vi "Day 4 Puzzle 1.vi"(11 "Path":path) -> ()   [LabVIEW 2021]
uses:
  <vilib>/Utility/file.llb/Read Delimited Spreadsheet (string).vi
panel:
  out "Number of contained":i32
  out "Array 4":bool[](array[boolean])
  out "Elf 2":i32[][](array[numeric])
  out "Elf 1":i32[][](array[numeric])
  out "subarray":string[](array[string])
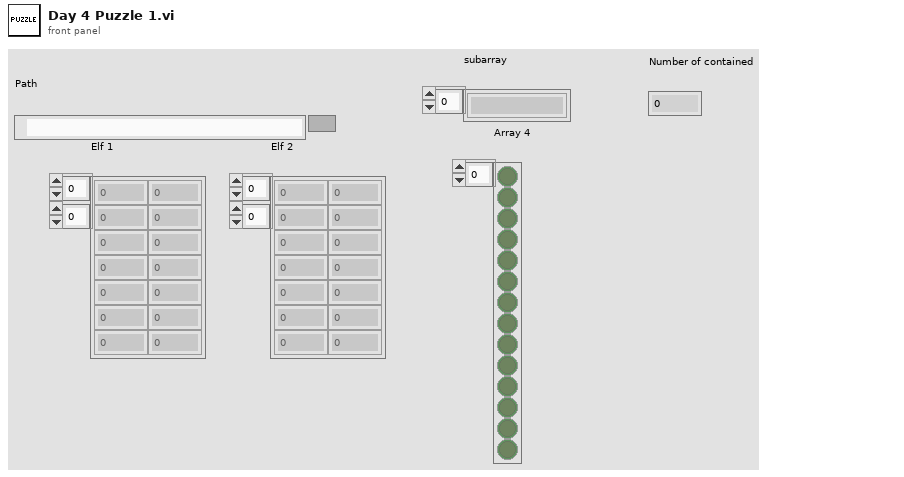
[diagram p1: front panel]
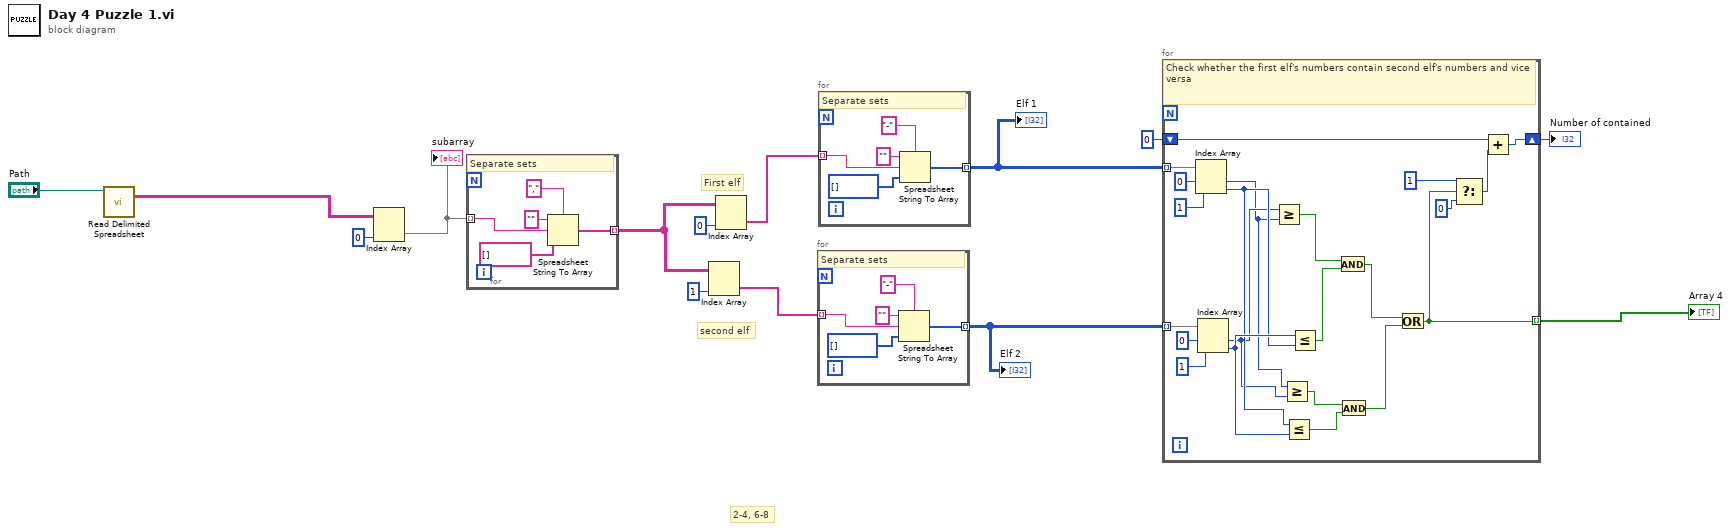
[diagram p0: block diagram]
diagram:
  # "2-4, 6-8"
  # "second elf"
  # "First elf"
  n1 = call-poly <vilib>:"Read Delimited Spreadsheet.vi"("file path (dialog if empty)"="Path") -> ("all rows"=w13:string[][])  [unwired: 9 in, 5 out]
  n2 = Index Array(array=w13, index (col)=0 ("disabled index (col)")) -> (element=w11:string[])  [unwired: 1 in]
  "subarray" <- w11
  n3 = for {
    tunnel: w11 -> [w17] mode=indexing
    tunnel: [w15] -> w8 mode=indexing
    # "Separate sets"
    n4 = Spreadsheet String To Array(delimiter (Tab)=",", format string="", spreadsheet string=w17, array type (2D Dbl)=string[] []) -> (array=w15:string[])
  }
  n5 = Index Array(array=w8, index (col)=1 ("disabled index (col)")) -> (element=w6:string[])  [unwired: 1 in]
  n6 = Index Array(array=w8, index (col)=0 ("disabled index (col)")) -> (element=w7:string[])  [unwired: 1 in]
  n7 = for {
    tunnel: w6 -> [w23] mode=indexing
    tunnel: [w21] -> w4 mode=indexing
    # "Separate sets"
    n8 = Spreadsheet String To Array(delimiter (Tab)="-", format string="", spreadsheet string=w23, array type (2D Dbl)=i32[] []) -> (array=w21:i32[])
  }
  "Elf 2" <- w4
  n9 = for {
    tunnel: w7 -> [w28] mode=indexing
    tunnel: [w26] -> w5 mode=indexing
    # "Separate sets"
    n10 = Spreadsheet String To Array(delimiter (Tab)="-", format string="", spreadsheet string=w28, array type (2D Dbl)=i32[] []) -> (array=w26:i32[])
  }
  "Elf 1" <- w5
  n11 = for {
    tunnel: w5 -> [w51] mode=indexing
    tunnel: w4 -> [w46] mode=indexing
    tunnel: [w35] -> w3 mode=indexing
    shift-right: [w31] -> w1
    shift-left: 0 -> [w34]
    # "Check whether the first elf's numbers contain second elf's numbers and vice versa"
    n12 = Index Array(array=w51, index #1=0 ("index"), index #2=1 ("index")) -> (element #1=w36:i32, element #2=w42:i32)
    n13 = Index Array(array=w46, index #1=0 ("index"), index #2=1 ("index")) -> (element #1=w37:i32, element #2=w43:i32)
    n14 = Greater Or Equal?(x=w37, y=w36) -> (x >= y?=w45:bool)
    n15 = Greater Or Equal?(x=w36, y=w37) -> (x >= y?=w40:bool)
    n16 = Less Or Equal?(x=w42, y=w43) -> (x <= y?=w41:bool)
    n17 = Less Or Equal?(x=w43, y=w42) -> (x <= y?=w44:bool)
    n18 = And(x=w45, y=w44) -> (x .and. y?=w39:bool)
    n19 = And(x=w40, y=w41) -> (x .and. y?=w38:bool)
    n20 = Or(x=w39, y=w38) -> (x .or. y?=w35:bool)
    n21 = Select(t=1, s=w35, f=0) -> (s? t:f=w33:i32)
    n22 = Add(x=w34, y=w33) -> (x+y=w31:i32)
  }
  "Array 4" <- w3
  "Number of contained" <- w1
